vi "LaserMaster.vi"() -> ()   [LabVIEW 2014]
uses:
  Serial/Serial.lvclass
  <vilib>/Utility/file.llb/Write To Spreadsheet File (string).vi
panel:
  out "Discovery?":bool
  out "Humidity Threshold":dbl
  in  "Power (mW) 2":dbl format="%#.0f"
  out "SavePath":path
  out "Start time":timestamp
  out "Step":dbl
  out "State next step":string
  in  "stop":bool
  out "Query backup List":string[][](array[string])=[["?L", " 0\r"], ["?K", " 0\r"], ["?F", " 0\r"], ["?FH", " 2\r"], ["?SHUTTER", " 0\r"], ["?UF", " 0\r"], ["?PHLDC", " 1\r"], ["?PZTMC", " 0\r"], ["?PZTXC", " 2.24\r"], ["?PZTYC", " 2.14\r"], ["?PHLDP", " 0\r"], ["?PZTMP", " 0\r"], ["?PZTXP", " 2.58\r"], ["?PXTYP", "  Query Error:?PXTYP\r"], ["?PTRK", "  Query Error:?PTRK\r"], ["?MDLK", " 0\r"], ["?PP", " 0.80\r"], ["?TS", " 0\r"], ["?SM", " 1\r"], ["?HM", " 1\r"], ["?VW", " 850\r"], ["?STPRPOS", " 2096\r"], ["?C", " 0.00\r"], ["?D1C", " 0.08\r"], ["?D2C", " -0.43\r"], ["?BT", " 20.07\r"], ["?D1T", " 24.20\r"], ["?D2T", " 24.20\r"], ["?VT", " 20.72\r"], ["?LBOT", " 148.45\r"], ["?ET", " 39.01\r"], ["?D1ST", " 24.20\r"], ["?D2ST", " 24.20\r"], ["?VST", " 30.00\r"], ["?LBOST", " 148.41\r"], ["?EST", " 39.00\r"], ["?D1TD", " 500.12\r"], ["?D2TD", " 464.53\r"], ["?VD", " 0.00\r"], ["?LBOD", " 5358.08\r"], ["?ED", " 2152.46\r"], ["?D1HST", " 21.35\r"], ["?D2HST", " 21.48\r"], ["?LBOH", " 1\r"], ["?LRS", " 2\r"], ["?D1SS", " 1\r"], ["?D2SS", " 1\r"], ["?VSS", " 0\r"], ["?LBOSS", " 1\r"], ["?ESS", " 1\r"], ["?D1H", "  351.54\r"], ["?D2H", "  351.52\r"], ["?HH", " 37\r"], ["?D1V", " 0.19\r"], ["?D2V", " 0.18\r"], ["?SV", " 8.26,8.26,9.57\r"], ["?MB", "  Query Error:?MB\r"], ["?PI", " 2BC\r"], ["?BV", " 13.24\r"], ["?AMDLK", " 1\r"], ["?PZTS", "  Query Error:?PZTS\r"], ["?TMAX", " 1080\r"], ["?TMIN", " 680\r"], ["?ALIGN", " 0\r"], ["?ALIGNP", " 250\r"], ["?ALIGNW", " 730\r"], ["?LFP", " 0\r"], ["?PZTXCM", " 8.11\r"], ["?PZTXCP", " -10.30\r"], ["?PZTXPM", " 8.11\r"], ["?PZTXPP", " 3.06\r"], ["?PZTYCM", " 8.11\r"], ["?PZTYCP", " -14.28\r"], ["?PZTYPM", " 8.11\r"], ["?PZTYPP", " 11.74\r"], ["?RH", " 0\r"], ["?SN", " 9571\r"], ["?ST", " Standby\r"], ["?GDDCURVE", " 0\r"], ["?GDD", " 0\r"], ["?GDDCURVEN", " ZERO\r"], ["?CURVEN", " OUT OF RANGE\r"], ["?COMP", " 1\r"], ["?HMCOMP", " 1\r"], ["?GDDMAX", " 17333\r"], ["?GDDMIN", "0"]]
  out "Laser Info":i32
  out "Shutter off time":dbl
  out "Quiting":dbl
  out "Backuper state":string
  in  "Tab Control":T1(tab)
  out "Power 2":i32
  in  "Align 2":bool
  in  "Shutter 2":bool
  in  "Lock":bool
  in  "Auto":bool
  out "Baseplate Temp (C)":dbl(slide) scale=20.0..40.0
  in  "Dither hold":bool
  in  "Shutter":bool
  out "Laser Status":bool
  out "Power (mW)":dbl(knob) scale=0.0..5000.0
  out "Walking":bool
  out "Sleeping":bool
  out "ModeLocked":bool
  out "Backing up":bool
  in  "Wavelength":dbl=920.0
  in  "GDD":dbl
  in  "QUIT":bool
  out "Max":string
  in  "Align":bool
  in  "Def. Wavelength":dbl=920.0
  in  "Dither auto":dbl=120.0
  in  "Dither timer":dbl=5.0
  out "Faults":string
  in  "Home motor":bool
  in  "Optimize":bool
  in  "WV Walk":bool
  in  "Standby Time (min)":dbl=120.0
  in  "Sleep":bool
  in  "Backup":bool
  in  "Auto-Backup \nIdle Time (min)":dbl=30.0
  out "Operating Status":string
  out "Tunning Status":i32
  out "Idle Time":dbl format="%.1f"
  out "Laser On Time":dbl format="%#.1f"
  in  "Laser Control":bool
  in  "Command Line":string
  out "Laser Response":string
  in  "Refresh":bool
  out "Query List":string[][](array[string])
  out "queue #":i32
  # "LASER"
  # "LASER fine-tune"
  # "BACKUP"
  # "Timers"
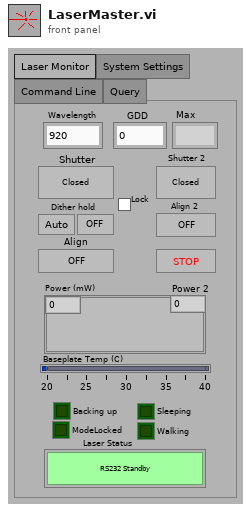
[diagram p1: front panel]
types:
  T1 = enum32{"Laser Monitor", "System Settings", "Command Line", "Query"}
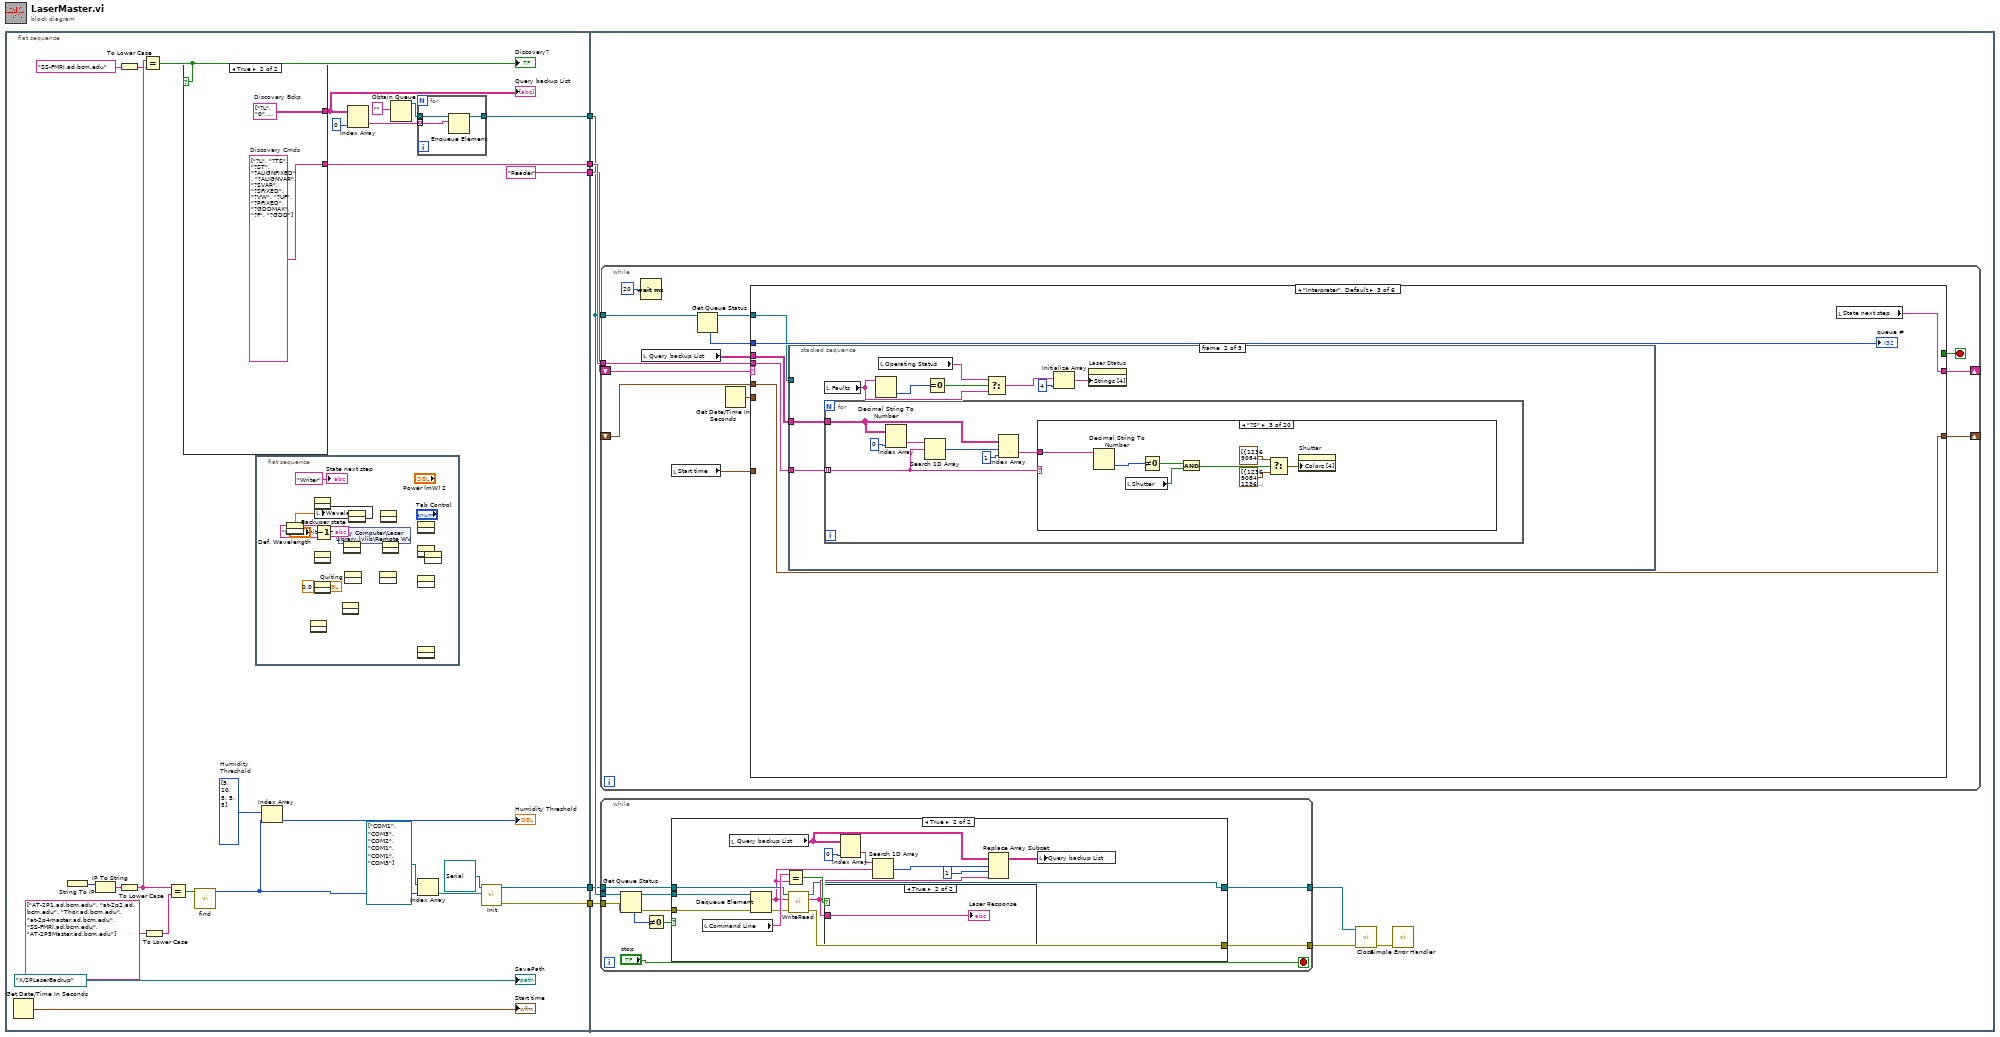
[diagram p0: block diagram]
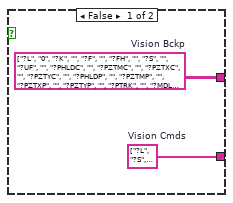
[diagram p2: hidden frame]
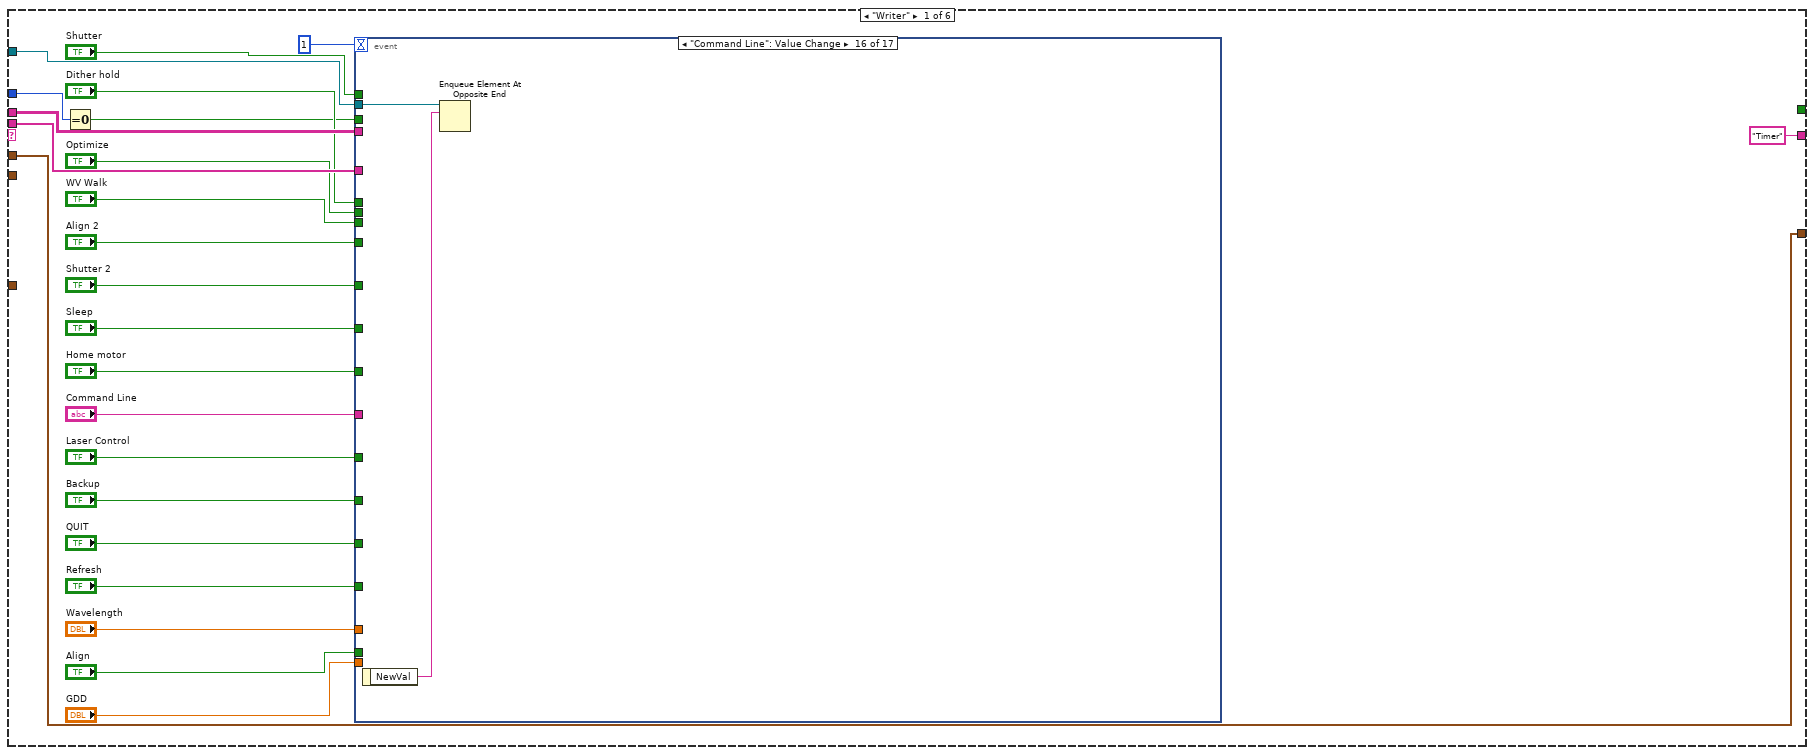
[diagram p5: hidden frame]
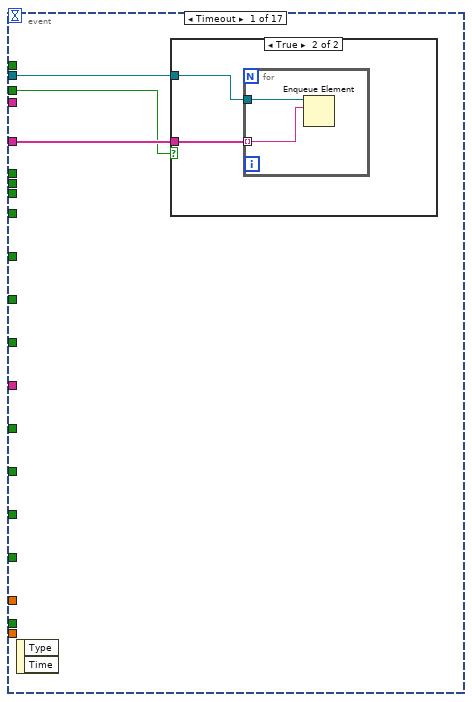
[diagram p6: hidden frame]
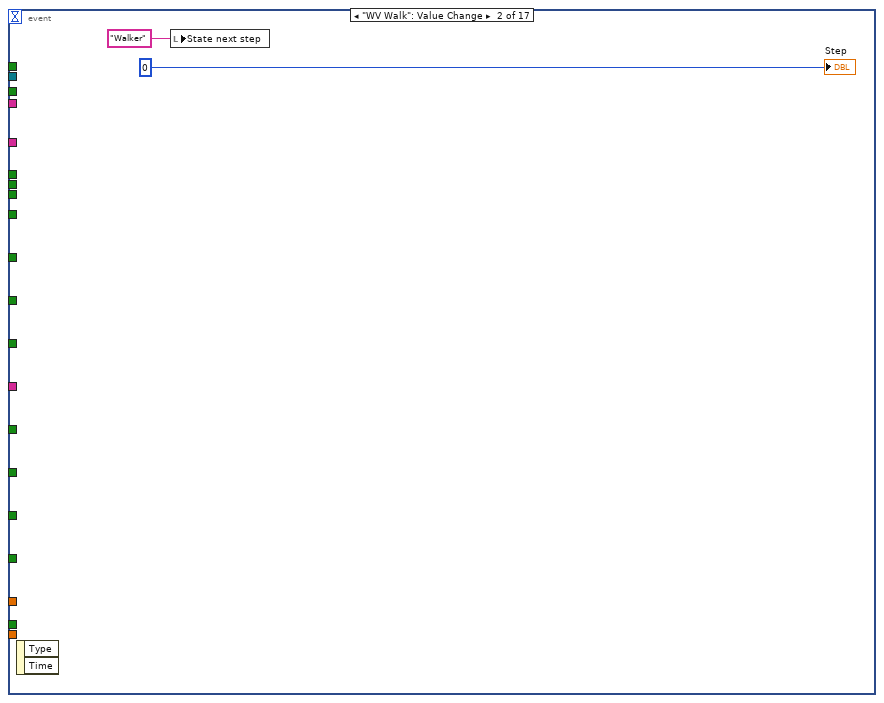
[diagram p8: hidden frame]
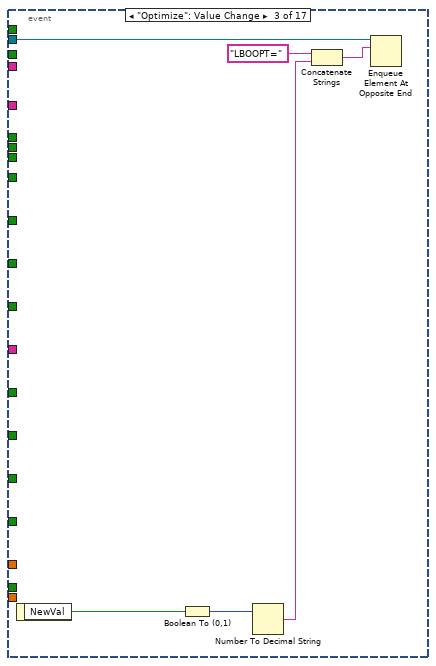
[diagram p9: hidden frame]
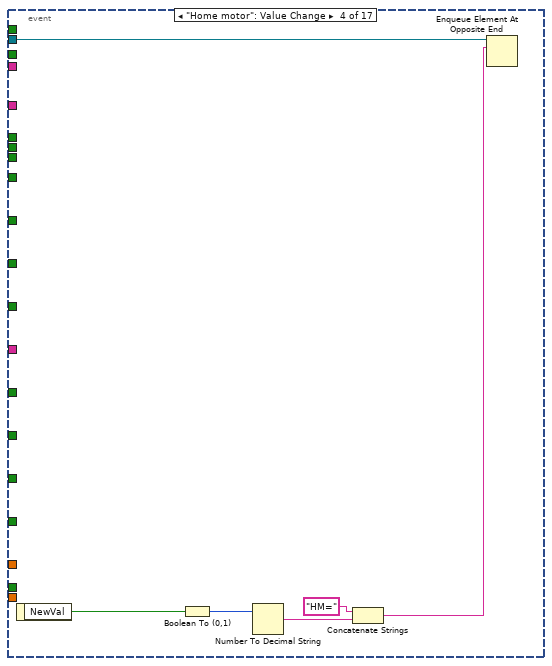
[diagram p10: hidden frame]
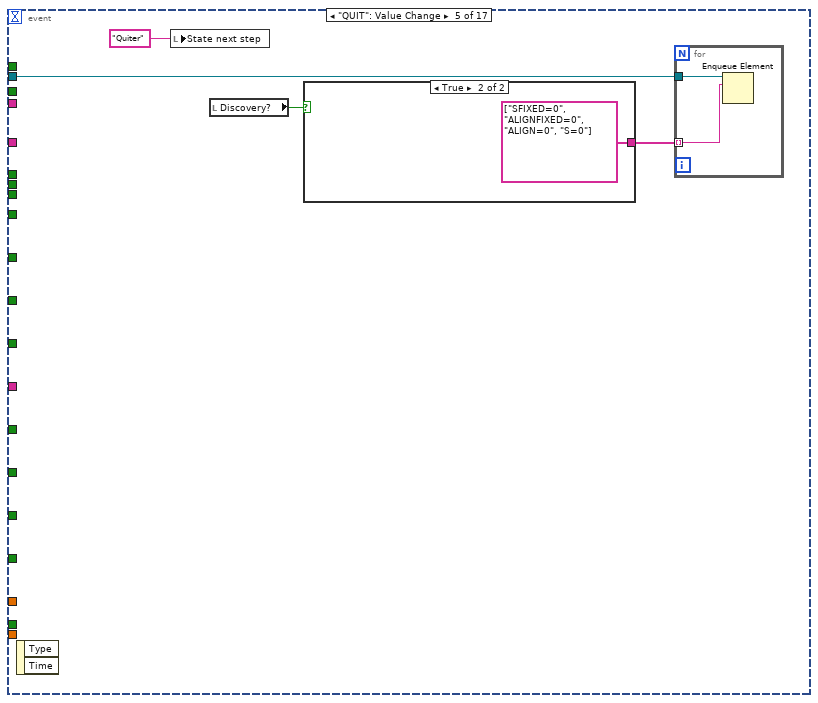
[diagram p11: hidden frame]
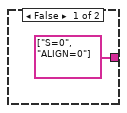
[diagram p12: hidden frame]
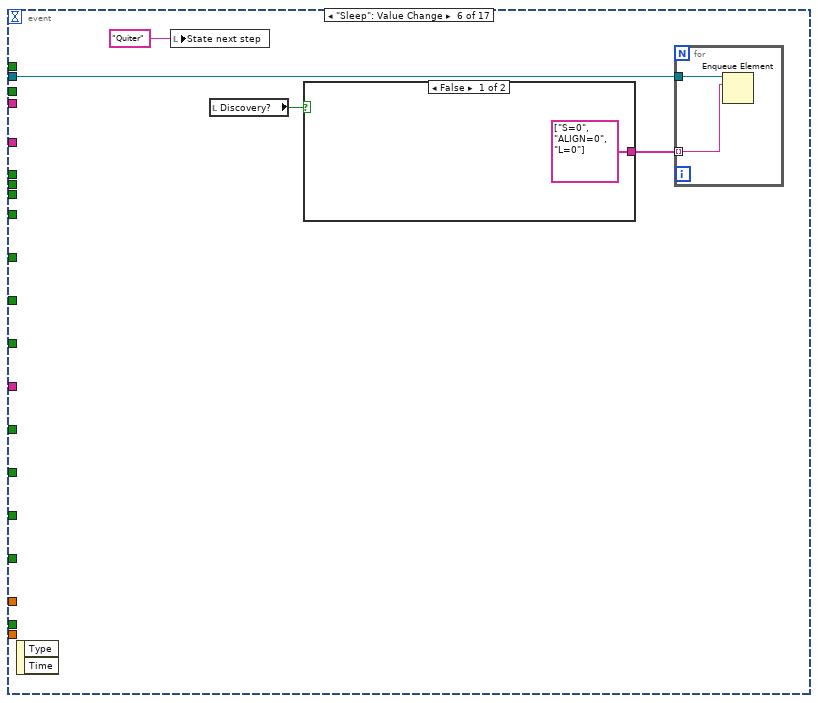
[diagram p13: hidden frame]
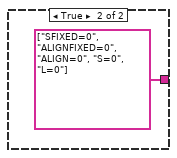
[diagram p14: hidden frame]
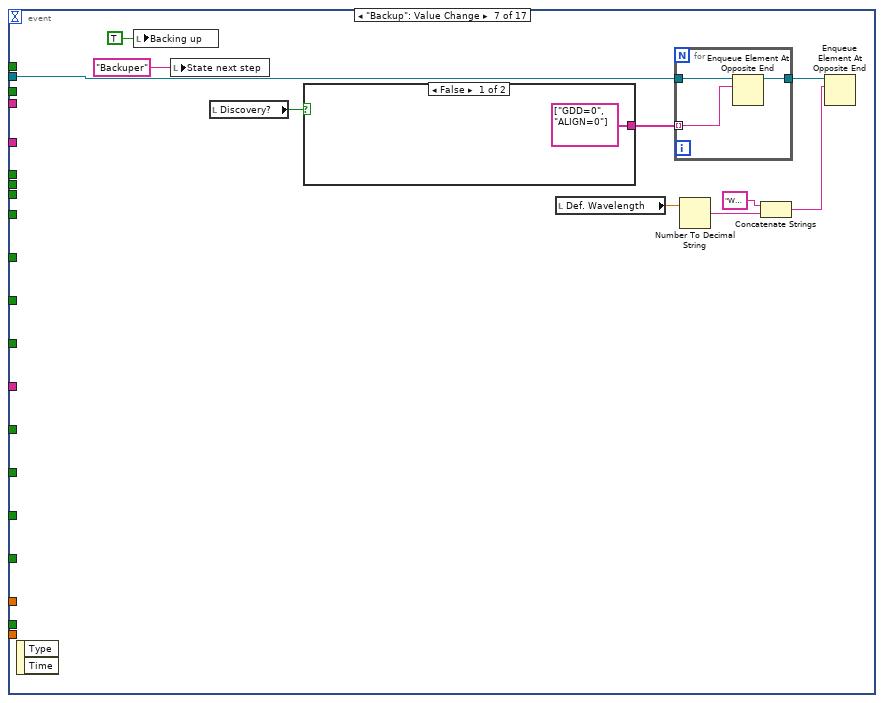
[diagram p15: hidden frame]
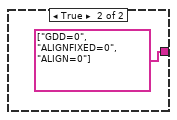
[diagram p16: hidden frame]
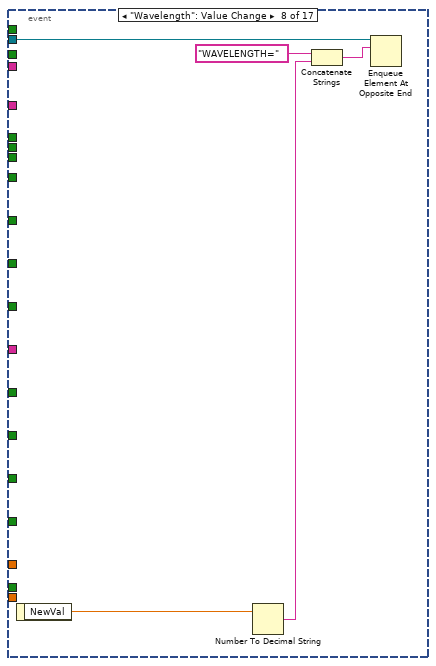
[diagram p17: hidden frame]
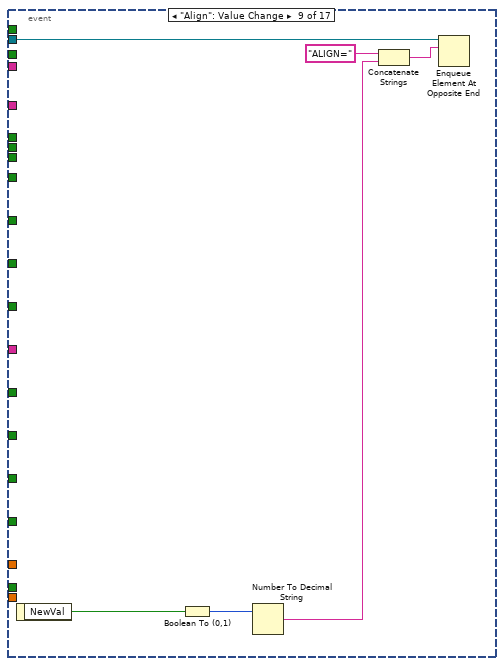
[diagram p18: hidden frame]
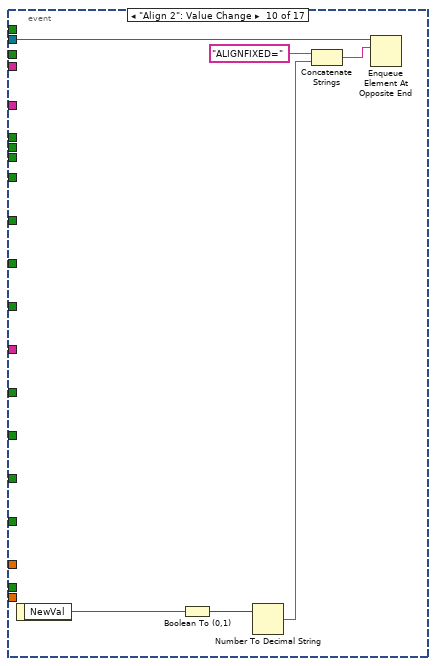
[diagram p19: hidden frame]
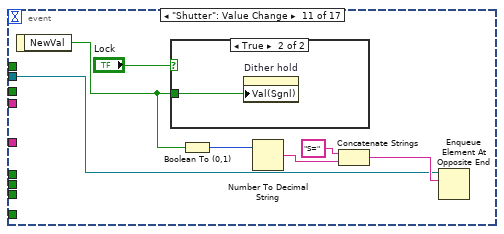
[diagram p20: hidden frame]
diagram:
  n1 = flat-sequence {
    tunnel: [w27] -> w5
    tunnel: [w10] -> w4
    tunnel: ["Reader"] -> w3
    tunnel: [w7] -> w2
    tunnel: [w6] -> w1
    tunnel: w5 -> [w50]
    tunnel: w4 -> [w52]
    tunnel: w3 -> [w51]
    tunnel: w2 -> [w49]
    tunnel: w1 -> [w48]
    frame #0 {
      w19 = i32[] [5, 10, 5, 5, 5]  # Humidity  Threshold
      n2 = Get Date/Time In Seconds() -> (seconds since 1Jan1904=→"Start time":timestamp)
      n3 = String To IP() -> (0:w24:u32)  [unwired: 1 in]
      n4 = IP To String(2:w24) -> (0:w22:string)  [unwired: 1 in]
      n5 = To Lower Case(string="SS-FMRI.ad.bcm.edu") -> (all lower case string=w13:string)
      n6 = To Lower Case(string=w22) -> (all lower case string=w15:string)
      n7 = Equal?(x=w15, y=w13) -> (x = y?=w12:bool)
      "Discovery?" <- w12
      n8 = To Lower Case(string=string[] ["AT-2P1.ad.bcm.edu", "at-2p2.ad.bcm.edu", "Thor.ad.bcm.edu", "at-2p4master.ad.bcm.edu", "SS-FMRI.ad.bcm.edu", "AT-2P5Master.ad.bcm.edu"]) -> (all lower case string=w23:string[])
      n9 = Equal?(x=w15, y=w23) -> (x = y?=w17:bool[])
      n10 = case shown="True" w12 {
        tunnel: [w34 w36] -> w11
        tunnel: [w33 w35] -> w10
        frame False {
          w33 = string[] ["?L", "?S", "?VW", "?ALIGN", "?PHLDP", "?UF", "?GDD", "?TS", "?ST", "?MDLK", "?GDDMAX", "?F", "?RH", "?BT"]  # Vision Cmds
          w34 = string[][] [["?L", "0"], ["?K", ""], ["?F", ""], ["?FH", ""], ["?S", ""], ["?UF", ""], ["?PHLDC", ""], ["?PZTMC", ""], ["?PZTXC", ""], ["?PZTYC", ""], ["?PHLDP", ""], ["?PZTMP", ""], ["?PZTXP", ""], ["?PZTYP", ""], ["?PTRK", ""], ["?MDLK", ""], ["?PP", ""], ["?TS", ""], ["?SM", ""], ["?HM", ""], ["?VW", ""], ["?STPRPOS", ""], ["?C", ""], ["?D1C", ""], ["?D2C", ""], ["?BT", ""], ["?D1T", ""], ["?D2T", ""], ["?VT", ""], ["?LBOT", ""], ["?ET", ""], ["?D1ST", ""], ["?D2ST", ""], ["?VST", ""], ["?LBOST", ""], ["?EST", ""], ["?D1TD", ""], ["?D2TD", ""], ["?VD", ""], ["?LBOD", ""], ["?ED", ""], ["?D1HST", ""], ["?D2HST", ""], ["?LBOH", ""], ["?LRS", ""], ["?D1SS", ""], ["?D2SS", ""], ["?VSS", ""], ["?LBOSS", ""], ["?ESS", ""], ["?D1H", ""], ["?D2H", ""], ["?HH", ""], ["?D1V", ""], ["?D2V", ""], ["?SV", ""], ["?PI", ""], ["?BV", ""], ["?AMDLK", ""], ["?PZTS", ""], ["?TMAX", ""], ["?TMIN", ""], ["?ALIGN", ""], ["?ALIGNP", ""], ["?ALIGNW", ""], ["?LFP", ""], ["?PZTXCM", ""], ["?PZTXCP", ""], ["?PZTXPM", ""], ["?PZTXPP", ""], ["?PZTYCM", ""], ["?PZTYCP", ""], ["?PZTYPM", ""], ["?PZTYPP", ""], ["?RH", ""], ["?SN", ""], ["?ST", ""], ["?GDDCURVE", ""], ["?GDD", ""], ["?GDDCURVEN", ""], ["?COMP", ""], ["?HMCOMP", ""], ["?GDDMAX", ""], ["?GDDMIN", ""]]  # Vision Bckp
        }
        frame True {
          w35 = string[] ["?L", "?TS", "?ST", "?ALIGNFIXED", "?ALIGNVAR", "?SVAR", "?SFIXED", "?VW", "?UF", "?PFIXED", "?GDDMAX", "?F", "?GDD"]  # Discovery Cmds
          w36 = string[][] [["?L", "0"], ["?K", ""], ["?TS", ""], ["?ST", ""], ["?ALIGNFIXED", ""], ["?ALIGNVAR", ""], ["?SVAR", ""], ["?SFIXED", ""], ["?VW", ""], ["?UF", ""], ["?PFIXED", ""], ["?HB", ""], ["?HRB", ""], ["?GDDCURVE", ""], ["?GDDCURVEN", ""], ["?GDD", ""], ["?GDDMAX", ""], ["?GDDMIN", ""], ["?SN", ""], ["?F", ""], ["?FT", ""], ["?FH", ""], ["?FHT", ""]]  # Discovery Bckp
        }
      }
      "Query backup List" <- w11
      n11 = call "find.vi"("Array"=w17) -> ("Index"=w16:i32)  [unwired: 10 in]
      n12 = flat-sequence {
        frame #0 {
          n13 = invoke on="ModeLocked" class="Bool (strict)" method="Reinit To Default"() -> ()  [unwired: 3 in, 3 out]
          n14 = invoke on="Align" class="Bool (strict)" method="Reinit To Default"() -> ()  [unwired: 3 in, 3 out]
          n15 = Decrement(x="Def. Wavelength") -> (x-1=w38:dbl)
          n16 = invoke on="Home motor" class="Bool" method="Reinit To Default"() -> ()  [unwired: 3 in, 3 out]
          n17 = invoke on="stop" class="Bool (strict)" method="Reinit To Default"() -> ()  [unwired: 3 in, 3 out]
          n18 = invoke on="Sleep" class="Bool (strict)" method="Reinit To Default"() -> ()  [unwired: 3 in, 3 out]
          n19 = local write "Wavelength"("Def. Wavelength") -> ()
          n20 = shared-variable "My Computer\\Laser Library.lvlib\\Remote WV"(w38) -> ()  [unwired: 1 in, 1 out]
          n21 = invoke on="WV Walk" class="Bool (strict)" method="Reinit To Default"() -> ()  [unwired: 3 in, 3 out]
          n22 = invoke on="Walking" class="Bool (strict)" method="Reinit To Default"() -> ()  [unwired: 3 in, 3 out]
          n23 = invoke on="Backup" class="Bool (strict)" method="Reinit To Default"() -> ()  [unwired: 3 in, 3 out]
          n24 = invoke on="Auto" class="Bool (strict)" method="Reinit To Default"() -> ()  [unwired: 3 in, 3 out]
          n25 = invoke on="Optimize" class="Bool" method="Reinit To Default"() -> ()  [unwired: 3 in, 3 out]
          n26 = invoke on="Sleeping" class="Bool (strict)" method="Reinit To Default"() -> ()  [unwired: 3 in, 3 out]
          n27 = invoke on="Refresh" class="Bool (strict)" method="Reinit To Default"() -> ()  [unwired: 3 in, 3 out]
          n28 = invoke on="Idle Time" class="DigNum (strict)" method="Reinit To Default"() -> ()  [unwired: 3 in, 3 out]
          n29 = invoke on="Laser Control" class="Bool (strict)" method="Reinit To Default"() -> ()  [unwired: 3 in, 3 out]
          n30 = invoke on="Dither hold" class="Bool (strict)" method="Reinit To Default"() -> ()  [unwired: 3 in, 3 out]
          n31 = invoke on="Backing up" class="Bool (strict)" method="Reinit To Default"() -> ()  [unwired: 3 in, 3 out]
          n32 = invoke on="QUIT" class="Bool (strict)" method="Reinit To Default"() -> ()  [unwired: 3 in, 3 out]
          "Backuper state" <- "BackupInit"
          "Quiting" <- 0.0 ("Quiting")
          "State next step" <- "Writer"
        }
      }
      n33 = Index Array(array=w19, index=w16) -> (element=→"Humidity Threshold":i32)
      n34 = Index Array(array=w11, index (col)=0 ("disabled index (col)")) -> (element=w29:string[])  [unwired: 1 in]
      n35 = Obtain Queue(element data type="") -> (queue out=w31:refnum<queue>)  [unwired: 4 in, 2 out]
      n36 = for {
        tunnel: w31 -> [w44]
        tunnel: w29 -> [w43] mode=indexing
        tunnel: [w42] -> w27
        n37 = Enqueue Element(queue=w44, element=w43) -> (queue out=w42:refnum<queue>)  [unwired: 2 in, 2 out]
      }
      n38 = Index Array(array=refnum<visa-resource-name>[] ["COM1", "COM3", "COM2", "COM1", "COM1", "COM3"], index=w16) -> (element=w9:refnum<visa-resource-name>)
      n39 = call-dynamic "Init.vi"("serial port"=w9, "Serial in"=refnum<class "Serial.lvclass"> refnum ("Serial.lvclass")) -> ("error out"=w6:errorcluster, "Serial out"=w7:refnum<class "Serial.lvclass">)  [unwired: 8 in]
      "SavePath" <- path "X:/2PLaserBackup"
    }
    frame #1 {
      n40 = while {
        tunnel: w50 -> [w91]
        tunnel: w52 -> [w92]
        shift-right: [w93] -> _
        shift-left: w51 -> [w94]
        shift-right: [w83] -> _
        shift-left: _ -> [w82]
        stop <- w88 stop-if-true
        n41 = Wait (ms)(milliseconds to wait=u32 20) -> ()  [unwired: 1 out]
        n42 = local read "Query backup List"() -> (w90:string[][])
        n43 = local read "Start time"() -> (w84:timestamp)
        n44 = Get Queue Status(queue=w91) -> (queue out=w87:refnum<queue>, # elements in queue=w86:i32)  [unwired: 2 in, 6 out]
        n45 = Get Date/Time In Seconds() -> (seconds since 1Jan1904=w85:timestamp)
        n46 = case shown="\"Interpreter\", Default" w94 {
          tunnel: w87 -> [w118 _ w298 _ _ _]
          tunnel: w90 -> [w117 _ w302 _ w495 _]
          tunnel: w92 -> [w116 _ w303 _ _ _]
          tunnel: ["Timer" "Interpreter" w301 "Writer" "Writer" w521] -> w93
          tunnel: w86 -> [w115 _ w300 _ _ w523]
          tunnel: [_ _ _ _ _ w520] -> w88
          tunnel: w85 -> [_ w232 _ _ _ _]
          tunnel: w84 -> [_ w236 _ _ _ _]
          tunnel: [w97 w233 w299 w477 w492 w519] -> w83
          tunnel: w82 -> [w97 w231 w299 w477 w492 w519]
          frame "Writer" {
            n47 = Equal To 0?(x=w115) -> (x = 0?=w103:bool)
            n48 = event shown="[15] \"Command Line\": Value Change" {
              selector: _ -> [_ _ _ _ _ _ _ _ _ _ _ _ _ _ _ _ _]
              dyn-events: _ -> [_ _ _ _ _ _ _ _ _ _ _ _ _ _ _ _ _]
              timeout: 1 -> [_ _ _ _ _ _ _ _ _ _ _ _ _ _ _ _ _]
              tunnel: w118 -> [w121 _ w128 w135 w143 w150 w165 w172 w177 w183 w190 w197 w203 w210 w215 w222 w224]
              tunnel: "Shutter" -> [_ _ _ _ _ _ _ _ _ _ _ _ _ _ _ _ _]
              tunnel: "Dither hold" -> [_ _ _ _ _ _ _ _ _ _ _ _ _ _ _ _ _]
              tunnel: "GDD" -> [_ _ _ _ _ _ _ _ _ _ _ _ _ _ _ _ _]
              tunnel: "Align" -> [_ _ _ _ _ _ _ _ _ _ _ _ _ _ _ _ _]
              tunnel: "Wavelength" -> [_ _ _ _ _ _ _ _ _ _ _ _ _ _ _ _ _]
              tunnel: "Laser Control" -> [_ _ _ _ _ _ _ _ _ _ _ _ _ _ _ _ _]
              tunnel: "Command Line" -> [_ _ _ _ _ _ _ _ _ _ _ _ _ _ _ _ _]
              tunnel: w117 -> [_ _ _ _ _ _ _ _ _ _ _ _ w202 _ _ _ _]
              tunnel: "Refresh" -> [_ _ _ _ _ _ _ _ _ _ _ _ _ _ _ _ _]
              tunnel: w116 -> [w120 _ _ _ _ _ _ _ _ _ _ _ _ _ _ _ _]
              tunnel: "QUIT" -> [_ _ _ _ _ _ _ _ _ _ _ _ _ _ _ _ _]
              tunnel: "Backup" -> [_ _ _ _ _ _ _ _ _ _ _ _ _ _ _ _ _]
              tunnel: w103 -> [w119 _ _ _ _ _ _ _ _ _ _ _ _ _ _ _ _]
              tunnel: "WV Walk" -> [_ _ _ _ _ _ _ _ _ _ _ _ _ _ _ _ _]
              tunnel: "Optimize" -> [_ _ _ _ _ _ _ _ _ _ _ _ _ _ _ _ _]
              tunnel: "Home motor" -> [_ _ _ _ _ _ _ _ _ _ _ _ _ _ _ _ _]
              tunnel: "Sleep" -> [_ _ _ _ _ _ _ _ _ _ _ _ _ _ _ _ _]
              tunnel: "Shutter 2" -> [_ _ _ _ _ _ _ _ _ _ _ _ _ _ _ _ _]
              tunnel: "Align 2" -> [_ _ _ _ _ _ _ _ _ _ _ _ _ _ _ _ _]
              event Timeout {
                n49 = event-data() -> ()  [unwired: 1 in, 2 out]
                n50 = case shown="True" w119 {
                  tunnel: w121 -> [_ w123]
                  tunnel: w120 -> [_ w122]
                  frame False {
                  }
                  frame True {
                    n51 = for {
                      tunnel: w123 -> [w125]
                      tunnel: w122 -> [w124] mode=indexing
                      n52 = Enqueue Element(queue=w125, element=w124) -> ()  [unwired: 2 in, 3 out]
                    }
                  }
                }
              }
              event "WV Walk": Value Change {
                n53 = event-data() -> ()  [unwired: 1 in, 2 out]
                n54 = local write "State next step"("Walker") -> ()
                "Step" <- 0
              }
              event "Optimize": Value Change {
                n55 = event-data() -> ("NewVal"=w129:bool)  [unwired: 1 in]
                n56 = Boolean To (0,1)(Boolean=w129) -> (0, 1=w132:i16)
                n57 = Number To Decimal String(number=w132) -> (decimal integer string=w133:string)  [unwired: 1 in]
                n58 = Concatenate Strings("LBOOPT=", w133) -> (w130:string)
                n59 = Enqueue Element At Opposite End(queue=w128, element=w130) -> ()  [unwired: 2 in, 3 out]
              }
              event "Home motor": Value Change {
                n60 = event-data() -> ("NewVal"=w134:bool)  [unwired: 1 in]
                n61 = Boolean To (0,1)(Boolean=w134) -> (0, 1=w138:i16)
                n62 = Number To Decimal String(number=w138) -> (decimal integer string=w139:string)  [unwired: 1 in]
                n63 = Concatenate Strings("HM=", w139) -> (w136:string)
                n64 = Enqueue Element At Opposite End(queue=w135, element=w136) -> ()  [unwired: 2 in, 3 out]
              }
              event "QUIT": Value Change {
                n65 = event-data() -> ()  [unwired: 1 in, 2 out]
                n66 = local write "State next step"("Quiter") -> ()
                n67 = local read "Discovery?"() -> (w140:bool)
                n68 = case shown="True" w140 {
                  tunnel: [string[] ["S=0", "ALIGN=0"] string[] ["SFIXED=0", "ALIGNFIXED=0", "ALIGN=0", "S=0"]] -> w141
                  frame False {
                  }
                  frame True {
                  }
                }
                n69 = for {
                  tunnel: w143 -> [w147]
                  tunnel: w141 -> [w146] mode=indexing
                  n70 = Enqueue Element(queue=w147, element=w146) -> ()  [unwired: 2 in, 3 out]
                }
              }
              event "Sleep": Value Change {
                n71 = event-data() -> ()  [unwired: 1 in, 2 out]
                n72 = local write "State next step"("Quiter") -> ()
                n73 = local read "Discovery?"() -> (w149:bool)
                n74 = case shown="False" w149 {
                  tunnel: [string[] ["S=0", "ALIGN=0", "L=0"] string[] ["SFIXED=0", "ALIGNFIXED=0", "ALIGN=0", "S=0", "L=0"]] -> w148
                  frame False {
                  }
                  frame True {
                  }
                }
                n75 = for {
                  tunnel: w150 -> [w155]
                  tunnel: w148 -> [w154] mode=indexing
                  n76 = Enqueue Element(queue=w155, element=w154) -> ()  [unwired: 2 in, 3 out]
                }
              }
              event "Backup": Value Change {
                n77 = event-data() -> ()  [unwired: 1 in, 2 out]
                n78 = local write "Backing up"(TRUE ("Backing up ...")) -> ()
                n79 = local write "State next step"("Backuper") -> ()
                n80 = local read "Discovery?"() -> (w157:bool)
                n81 = case shown="False" w157 {
                  tunnel: [string[] ["GDD=0", "ALIGN=0"] string[] ["GDD=0", "ALIGNFIXED=0", "ALIGN=0"]] -> w156
                  frame False {
                  }
                  frame True {
                  }
                }
                n82 = local read "Def. Wavelength"() -> (w161:dbl)
                n83 = for {
                  tunnel: w156 -> [w170] mode=indexing
                  tunnel: w165 -> [w169]
                  tunnel: [w168] -> w162
                  n84 = Enqueue Element At Opposite End(queue=w169, element=w170) -> (queue out=w168:refnum<queue>)  [unwired: 2 in, 2 out]
                }
                n85 = Number To Decimal String(number=w161) -> (decimal integer string=w159:string)  [unwired: 1 in]
                n86 = Concatenate Strings("WAVELENGTH=", w159) -> (w158:string)
                n87 = Enqueue Element At Opposite End(queue=w162, element=w158) -> ()  [unwired: 2 in, 3 out]
              }
              event "Wavelength": Value Change {
                n88 = event-data() -> ("NewVal"=w171:dbl)  [unwired: 1 in]
                n89 = Number To Decimal String(number=w171) -> (decimal integer string=w174:string)  [unwired: 1 in]
                n90 = Concatenate Strings("WAVELENGTH=", w174) -> (w175:string)
                n91 = Enqueue Element At Opposite End(queue=w172, element=w175) -> ()  [unwired: 2 in, 3 out]
              }
              event "Align": Value Change {
                n92 = event-data() -> ("NewVal"=w176:bool)  [unwired: 1 in]
                n93 = Boolean To (0,1)(Boolean=w176) -> (0, 1=w180:i16)
                n94 = Number To Decimal String(number=w180) -> (decimal integer string=w181:string)  [unwired: 1 in]
                n95 = Concatenate Strings("ALIGN=", w181) -> (w178:string)
                n96 = Enqueue Element At Opposite End(queue=w177, element=w178) -> ()  [unwired: 2 in, 3 out]
              }
              event "Align 2": Value Change {
                n97 = event-data() -> ("NewVal"=w182:bool)  [unwired: 1 in]
                n98 = Boolean To (0,1)(Boolean=w182) -> (0, 1=w186:i16)
                n99 = Number To Decimal String(number=w186) -> (decimal integer string=w187:string)  [unwired: 1 in]
                n100 = Concatenate Strings("ALIGNFIXED=", w187) -> (w184:string)
                n101 = Enqueue Element At Opposite End(queue=w183, element=w184) -> ()  [unwired: 2 in, 3 out]
              }
              event "Shutter": Value Change {
                n102 = event-data() -> ("NewVal"=w188:bool)  [unwired: 1 in]
                n103 = case shown="True" "Lock" {
                  tunnel: w188 -> [_ w195]
                  frame False {
                  }
                  frame True {
                    n104 = property on="Dither hold" class="Bool (strict)"("Val(Sgnl)"=w195) -> ()  [unwired: 2 in, 2 out]
                  }
                }
                n105 = Boolean To (0,1)(Boolean=w188) -> (0, 1=w193:i16)
                n106 = Number To Decimal String(number=w193) -> (decimal integer string=w194:string)  [unwired: 1 in]
                n107 = Concatenate Strings("S=", w194) -> (w191:string)
                n108 = Enqueue Element At Opposite End(queue=w190, element=w191) -> ()  [unwired: 2 in, 3 out]
              }
              event "Shutter 2": Value Change {
                n109 = event-data() -> ("NewVal"=w196:bool)  [unwired: 1 in]
                n110 = Boolean To (0,1)(Boolean=w196) -> (0, 1=w200:i16)
                n111 = Number To Decimal String(number=w200) -> (decimal integer string=w201:string)  [unwired: 1 in]
                n112 = Concatenate Strings("SFIXED=", w201) -> (w198:string)
                n113 = Enqueue Element At Opposite End(queue=w197, element=w198) -> ()  [unwired: 2 in, 3 out]
              }
              event "Refresh": Value Change {
                n114 = event-data() -> ()  [unwired: 1 in, 1 out]
                n115 = local write "Refresh"(FALSE ("Backup")) -> ()
                n116 = Index Array(array=w202, index (col)=0 ("disabled index (col)")) -> (element=w205:string[])  [unwired: 1 in]
                n117 = for {
                  tunnel: w203 -> [w208]
                  tunnel: w205 -> [w207] mode=indexing
                  n118 = Enqueue Element(queue=w208, element=w207) -> ()  [unwired: 2 in, 3 out]
                }
              }
              event "Dither hold": Value Change {
                n119 = event-data() -> ("NewVal"=w209:bool)  [unwired: 1 in]
                n120 = Boolean To (0,1)(Boolean=w209) -> (0, 1=w213:i16)
                n121 = Number To Decimal String(number=w213) -> (decimal integer string=w214:string)  [unwired: 1 in]
                n122 = Concatenate Strings("PHLDP=", w214) -> (w211:string)
                n123 = Enqueue Element At Opposite End(queue=w210, element=w211) -> ()  [unwired: 2 in, 3 out]
              }
              event "Laser Control": Value Change {
                n124 = event-data() -> ("NewVal"=w216:bool)  [unwired: 1 in]
                n125 = Boolean To (0,1)(Boolean=w216) -> (0, 1=w219:i16)
                n126 = Number To Decimal String(number=w219) -> (decimal integer string=w220:string)  [unwired: 1 in]
                n127 = Concatenate Strings("L=", w220) -> (w217:string)
                n128 = Enqueue Element At Opposite End(queue=w215, element=w217) -> ()  [unwired: 2 in, 3 out]
              }
              event "Command Line": Value Change {
                n129 = event-data() -> ("NewVal"=w221:string)  [unwired: 1 in]
                n130 = Enqueue Element At Opposite End(queue=w222, element=w221) -> ()  [unwired: 2 in, 3 out]
              }
              event "GDD": Value Change {
                n131 = event-data() -> ("NewVal"=w223:dbl)  [unwired: 1 in]
                n132 = Number To Decimal String(number=w223) -> (decimal integer string=w226:string)  [unwired: 1 in]
                n133 = Concatenate Strings("GDD=", w226) -> (w227:string)
                n134 = Enqueue Element At Opposite End(queue=w224, element=w227) -> ()  [unwired: 2 in, 3 out]
              }
            }
          }
          frame "Timer" {
            n135 = Subtract(x=w232, y=w236) -> (x-y=w239:dbl)
            n136 = local read "Tunning Status"() -> (w256:i32)
            n137 = local read "Laser Control"() -> (w255:bool)
            n138 = local read "Power (mW)"() -> (w229:dbl)
            n139 = case shown="True" "Auto" {
              tunnel: w232 -> [w258 w265]
              tunnel: [w258 w264] -> w233
              tunnel: w231 -> [_ w263]
              frame False {
              }
              frame True {
                n140 = Subtract(x=w265, y=w263) -> (x-y=w267:dbl)
                n141 = local read "Dither hold"() -> (w259:bool)
                n142 = Select(t="Dither auto", s=w259, f="Dither timer") -> (s? t:f=w260:dbl)
                n143 = Greater?(x=w267, y=w260) -> (0:w266:bool)
                n144 = case shown="True" w266 {
                  tunnel: w265 -> [_ w271]
                  tunnel: [w268 w271] -> w264
                  tunnel: w263 -> [w268 _]
                  tunnel: w259 -> [_ w270]
                  frame False {
                  }
                  frame True {
                    n145 = Not(x=w270) -> (.not. x?=w269:bool)
                    n146 = property on="Dither hold" class="Bool (strict)"("Val(Sgnl)"=w269) -> ()  [unwired: 2 in, 2 out]
                  }
                }
              }
            }
            n147 = Not(x=w255) -> (.not. x?=w251:bool)
            n148 = Equal To 0?(x=w256) -> (x = 0?=w250:bool)
            n149 = Less?(x=w229, y=1.0) -> (x < y?=w228:bool)
            n150 = local read "Shutter off time"() -> (w246:dbl)
            n151 = local read "Shutter"() -> (w247:bool)
            n152 = Compound Arithmetic op=AND(w228, w251, w250) -> (w252:bool)
            n153 = Divide(x=w239, y=60.0 ("x")) -> (x/y=w237:dbl)
            n154 = case shown="False" w252 {
              tunnel: [w272 w283] -> w249
              tunnel: [w276 w283] -> w248
              tunnel: w247 -> [w275 _]
              tunnel: w246 -> [w274 _]
              tunnel: [w273 w283] -> w245
              tunnel: w237 -> [w272 _]
              frame False {
                n155 = case shown="False" w275 {
                  tunnel: [w279 0] -> w276
                  tunnel: w272 -> [w278 w280]
                  tunnel: w274 -> [w277 _]
                  tunnel: [w277 w280] -> w273
                  frame False {
                    n156 = Subtract(x=w278, y=w277) -> (x-y=w279:dbl)
                  }
                  frame True {
                  }
                }
              }
              frame True {
                w283 = 0
                n157 = Get Date/Time In Seconds() -> (seconds since 1Jan1904=w282:timestamp)
                n158 = local write "Start time"(w282) -> ()
              }
            }
            "Laser On Time" <- w249
            "Idle Time" <- w248
            "Shutter off time" <- w245
            n159 = local read "Backing up"() -> (w240:bool)
            n160 = Greater?(x=w248, y="Auto-Backup \nIdle Time (min)") -> (0:w243:bool)
            n161 = Greater?(x=w248, y="Standby Time (min)") -> (0:w235:bool)
            n162 = Not(x=w240) -> (.not. x?=w242:bool)
            n163 = case shown="True" w235 {
              tunnel: [FALSE ("Sleeping") w285] -> w244
              frame False {
              }
              frame True {
                w285 = TRUE
                n164 = property on="Sleep" class="Bool (strict)"("Val(Sgnl)"=w285) -> ()  [unwired: 2 in, 2 out]
              }
            }
            "Sleeping" <- w244
            n165 = And(x=w243, y=w242) -> (x .and. y?=w241:bool)
            n166 = case shown="True" w241 {
              frame False {
              }
              frame True {
                n167 = Get Date/Time In Seconds() -> (seconds since 1Jan1904=w292:timestamp)
                n168 = Format Date/Time String(time format string (%c)="%Y-%m-%d-*", seconds (now)=w292) -> (date/time string=w289:string)  [unwired: 1 in]
                n169 = String To IP() -> (0:w290:u32)  [unwired: 1 in]
                n170 = local read "SavePath"() -> (w286:path)
                n171 = IP To String(2:w290) -> (0:w287:string)  [unwired: 1 in]
                n172 = Concatenate Strings(w289, ".csv" ("string")) -> (w294:string)
                n173 = call "create unique folder.vi"("string"=w287, "path 2"=w286) -> ("path"=w295:path)  [unwired: 9 in]
                n174 = call <vilib>:"Recursive File List.vi"("pattern"=w294, "Folder Path"=w295) -> ("Number of Files"=w296:i32)  [unwired: 5 in, 4 out]
                n175 = Equal To 0?(x=w296) -> (x = 0?=w288:bool)
                n176 = case shown="True" w288 {
                  frame False {
                  }
                  frame True {
                    n177 = property on="Backup" class="Bool (strict)"("Val(Sgnl)"=TRUE) -> ()  [unwired: 2 in, 2 out]
                  }
                }
              }
            }
          }
          frame "Interpreter", Default {
            n178 = stacked-sequence {
              tunnel: w303 -> [_ w318 _ _ _]
              tunnel: w302 -> [_ w317 _ w442 _]
              tunnel: w298 -> [w304 _ _ _ _]
              frame #0 {
                n179 = local read "Command Line"() -> (w306:string)
                n180 = feedback-in #1(w306) -> ()
                n181 = feedback #1() -> (w307:string)  [unwired: 1 in]
                n182 = Not Equal?(x=w307, y=w306) -> (x != y?=w305:bool)
                n183 = case shown="True" w305 {
                  tunnel: w304 -> [_ w309]
                  tunnel: w306 -> [_ w308]
                  frame False {
                  }
                  frame True {
                    n184 = Enqueue Element At Opposite End(queue=w309, element=w308) -> ()  [unwired: 2 in, 3 out]
                  }
                }
              }
              frame #1 {
                n185 = local read "Faults"() -> (w311:string)
                n186 = for {
                  tunnel: w318 -> [w320] mode=indexing
                  tunnel: w317 -> [w321]
                  n187 = Index Array(array=w321, index (col)=0 ("disabled index (col)")) -> (element=w324:string[])  [unwired: 1 in]
                  n188 = Search 1D Array(1D array=w324, element=w320) -> (index of element=w322:i32)  [unwired: 1 in]
                  n189 = Index Array(array=w321, index (row)=w322, index (col)=1 ("disabled index (col)")) -> (element=w319:string)
                  n190 = case shown="\"?S\"" w320 {
                    tunnel: w319 -> [_ w326 w332 w337 w342 w350 w358 w366 w374 w378 w387 w390 w392 w400 w402 w404 w406 w407 w418 w420]
                    frame "False", Default {
                    }
                    frame "?L" {
                      n191 = Decimal String To Number(string=w326) -> (number=→"Laser Info":i32)  [unwired: 2 in, 1 out]
                    }
                    frame "?S" {
                      n192 = Decimal String To Number(string=w332) -> (number=w333:i32)  [unwired: 2 in, 1 out]
                      n193 = local read "Shutter"() -> (w335:bool)
                      n194 = Not Equal To 0?(x=w333) -> (x != 0?=w334:bool)
                      n195 = And(x=w334, y=w335) -> (x .and. y?=w328:bool)
                      n196 = Select(t=cluster{u32, u32}[] [{12369084, 12369084}, {6618880, 6618880}] ("Colors [4]"), s=w328, f=cluster{u32, u32}[] [{12369084, 12369084}, {12369084, 12369084}] ("Colors [4]")) -> (s? t:f=w329:cluster{u32, u32}[])
                      n197 = property on="Shutter" class="Bool (strict)"("Colors [4]"=w329) -> ()  [unwired: 2 in, 2 out]
                    }
                    frame "?VW" {
                      n198 = Decimal String To Number(string=w337) -> (number=w336:i32)  [unwired: 2 in, 1 out]
                      n199 = property on="Wavelength" class="DigNum (strict)"("Value"=w336) -> ()  [unwired: 2 in, 2 out]
                      n200 = shared-variable ".\\Laser Library.lvlib\\WV"(w336) -> ()  [unwired: 1 in, 1 out]
                    }
                    frame "?SVAR" {
                      n201 = Decimal String To Number(string=w342) -> (number=w343:i32)  [unwired: 2 in, 1 out]
                      n202 = local read "Shutter"() -> (w345:bool)
                      n203 = Not Equal To 0?(x=w343) -> (x != 0?=w344:bool)
                      n204 = And(x=w344, y=w345) -> (x .and. y?=w338:bool)
                      n205 = Select(t=cluster{u32, u32}[] [{12369084, 12369084}, {6618880, 6618880}] ("Colors [4]"), s=w338, f=cluster{u32, u32}[] [{12369084, 12369084}, {12369084, 12369084}] ("Colors [4]")) -> (s? t:f=w339:cluster{u32, u32}[])
                      n206 = property on="Shutter" class="Bool (strict)"("Colors [4]"=w339) -> ()  [unwired: 2 in, 2 out]
                    }
                    frame "?SFIXED" {
                      n207 = Decimal String To Number(string=w350) -> (number=w351:i32)  [unwired: 2 in, 1 out]
                      n208 = local read "Shutter 2"() -> (w353:bool)
                      n209 = Not Equal To 0?(x=w351) -> (x != 0?=w352:bool)
                      n210 = And(x=w352, y=w353) -> (x .and. y?=w346:bool)
                      n211 = Select(t=cluster{u32, u32}[] [{12369084, 12369084}, {6618880, 6618880}] ("Colors [4]"), s=w346, f=cluster{u32, u32}[] [{12369084, 12369084}, {12369084, 12369084}] ("Colors [4]")) -> (s? t:f=w349:cluster{u32, u32}[])
                      n212 = property on="Shutter 2" class="Bool (strict)"("Colors [4]"=w349) -> ()  [unwired: 2 in, 2 out]
                    }
                    frame "?ALIGN" {
                      n213 = Decimal String To Number(string=w358) -> (number=w359:i32)  [unwired: 2 in, 1 out]
                      n214 = Not Equal To 0?(x=w359) -> (x != 0?=w361:bool)
                      n215 = local read "Align"() -> (w360:bool)
                      n216 = And(x=w361, y=w360) -> (x .and. y?=w355:bool)
                      n217 = Select(t=cluster{u32, u32}[] [{12369084, 12369084}, {6618880, 6618880}] ("Colors [4]"), s=w355, f=cluster{u32, u32}[] [{12369084, 12369084}, {12369084, 12369084}] ("Colors [4]")) -> (s? t:f=w354:cluster{u32, u32}[])
                      n218 = property on="Align" class="Bool (strict)"("Colors [4]"=w354) -> ()  [unwired: 2 in, 2 out]
                    }
                    frame "?ALIGNVAR" {
                      n219 = Decimal String To Number(string=w366) -> (number=w367:i32)  [unwired: 2 in, 1 out]
                      n220 = Not Equal To 0?(x=w367) -> (x != 0?=w369:bool)
                      n221 = local read "Align"() -> (w368:bool)
                      n222 = And(x=w369, y=w368) -> (x .and. y?=w362:bool)
                      n223 = Select(t=cluster{u32, u32}[] [{12369084, 12369084}, {6618880, 6618880}] ("Colors [4]"), s=w362, f=cluster{u32, u32}[] [{12369084, 12369084}, {12369084, 12369084}] ("Colors [4]")) -> (s? t:f=w363:cluster{u32, u32}[])
                      n224 = property on="Align" class="Bool (strict)"("Colors [4]"=w363) -> ()  [unwired: 2 in, 2 out]
                    }
                    frame "?ALIGNFIXED" {
                      n225 = Decimal String To Number(string=w374) -> (number=w375:i32)  [unwired: 2 in, 1 out]
                      n226 = local read "Align 2"() -> (w376:bool)
                      n227 = Not Equal To 0?(x=w375) -> (x != 0?=w377:bool)
                      n228 = And(x=w377, y=w376) -> (x .and. y?=w371:bool)
                      n229 = Select(t=cluster{u32, u32}[] [{12369084, 12369084}, {6618880, 6618880}] ("Colors [4]"), s=w371, f=cluster{u32, u32}[] [{12369084, 12369084}, {12369084, 12369084}] ("Colors [4]")) -> (s? t:f=w372:cluster{u32, u32}[])
                      n230 = property on="Align 2" class="Bool (strict)"("Colors [4]"=w372) -> ()  [unwired: 2 in, 2 out]
                    }
                    frame "?PHLDP" {
                      n231 = Decimal String To Number(string=w378) -> (number=w379:i32)  [unwired: 2 in, 1 out]
                      n232 = Not Equal To 0?(x=w379) -> (x != 0?=w382:bool)
                      n233 = local read "Dither hold"() -> (w380:bool)
                      n234 = And(x=w382, y=w380) -> (x .and. y?=w381:bool)
                      n235 = case shown="False" w381 {
                        frame False {
                          n236 = property on="Dither hold" class="Bool (strict)"("Colors [4]"=cluster{u32, u32}[] [{12369084, 12369084}, {12369084, 12369084}]) -> ()  [unwired: 2 in, 2 out]
                        }
                        frame True {
                          n237 = property on="Dither hold" class="Bool (strict)"("Colors [4]"=cluster{u32, u32}[] [{12369084, 12369084}, {6618880, 6618880}]) -> ()  [unwired: 2 in, 2 out]
                        }
                      }
                    }
                    frame "?UF" {
                      n238 = Decimal String To Number(string=w387) -> (number=w386:i32)  [unwired: 2 in, 1 out]
                      n239 = Round To Nearest(number=w386) -> (nearest integer value=→"Power (mW)":i32)
                    }
                    frame "?PFIXED" {
                      n240 = Decimal String To Number(string=w390) -> (number=w389:i32)  [unwired: 2 in, 1 out]
                      n241 = Round To Nearest(number=w389) -> (nearest integer value=→"Power 2":i32)
                    }
                    frame "?GDD" {
                      n242 = Decimal String To Number(string=w392) -> (number=w391:i32)  [unwired: 2 in, 1 out]
                      n243 = property on="GDD" class="DigNum (strict)"("Value"=w391) -> ()  [unwired: 2 in, 2 out]
                      n244 = shared-variable "My Computer\\Laser Library.lvlib\\GDD"(w391) -> ()  [unwired: 1 in, 1 out]
                    }
                    frame "?GDDMAX" {
                      n245 = Decimal String To Number(string=w400) -> (number=w398:i32)  [unwired: 2 in, 1 out]
                      n246 = Divide(x=w398, y=1000.0) -> (x/y=w394:dbl)
                      n247 = Round To Nearest(number=w394) -> (nearest integer value=w393:dbl)
                      n248 = Number To Decimal String(number=w393) -> (decimal integer string=w397:string)  [unwired: 1 in]
                      n249 = Concatenate Strings(w397, "k" ("string")) -> (→"Max":string)
                    }
                    frame "?TS" {
                      n250 = Decimal String To Number(string=w402) -> (number=→"Tunning Status":i32)  [unwired: 2 in, 1 out]
                    }
                    frame "?MDLK" {
                      n251 = Decimal String To Number(string=w404) -> (number=w405:i32)  [unwired: 2 in, 1 out]
                      n252 = Not Equal To 0?(x=w405) -> (x != 0?=→"ModeLocked":bool)
                    }
                    frame "?ST" {
                      "Operating Status" <- w406
                    }
                    frame "?F" {
                      "Faults" <- w407
                    }
                    frame "?RH" {
                      n253 = Decimal String To Number(string=w418) -> (number=w417:i32)  [unwired: 2 in, 1 out]
                      n254 = local read "Humidity Threshold"() -> (w408:dbl)
                      n255 = local read "Operating Status"() -> (w411:string)
                      n256 = local read "Laser Info"() -> (w414:i32)
                      n257 = Concatenate Strings(w411, "\nHigh Humidity") -> (w409:string)
                      n258 = Greater?(x=w417, y=w408) -> (0:w416:bool)
                      n259 = Select(t=w409, s=w416, f=w411) -> (s? t:f=w412:string)
                      n260 = Select(t=2, s=w416, f=w414) -> (s? t:f=w415:i32)
                      n261 = local write "Operating Status"(w412) -> ()
                      n262 = local write "Laser Info"(w415) -> ()
                    }
                    frame "?BT" {
                      n263 = Decimal String To Number(string=w420) -> (number=→"Baseplate Temp (C)":i32)  [unwired: 2 in, 1 out]
                    }
                  }
                }
                n264 = Decimal String To Number(string=w311) -> (number=w312:i32)  [unwired: 2 in, 1 out]
                n265 = local read "Operating Status"() -> (w313:string)
                n266 = Equal To 0?(x=w312) -> (x = 0?=w310:bool)
                n267 = Select(t=w313, s=w310, f=w311) -> (s? t:f=w314:string)
                n268 = Initialize Array(w314, 4 ("dimension size")) -> (w315:string[])
                n269 = property on="Laser Status" class="Bool (strict)"("Strings [4]"=w315) -> ()  [unwired: 2 in, 2 out]
              }
              frame #2 {
                n270 = local read "Tunning Status"() -> (w425:i32)
                n271 = local read "Laser Info"() -> (w423:i32)
                n272 = Equal To 0?(x=w425) -> (x = 0?=w426:bool)
                n273 = Equal To 0?(x=w423) -> (x = 0?=w422:bool)
                n274 = And(x=w426, y=w422) -> (x .and. y?=w424:bool)
                n275 = Equal?(x=w423, y=2.0) -> (x = y?=w428:bool)
                n276 = case shown="False" w428 {
                  tunnel: w424 -> [w430 _]
                  tunnel: [w429 cluster{u32, u32}[] [{16723218, 15670016}, {16721170, 16725034}] ("Colors [4]")] -> w421
                  frame False {
                    n277 = case shown="False" w430 {
                      tunnel: [w431 cluster{u32, u32}[] [{10682272, 10682272}, {12451729, 12451729}] ("Colors [4]")] -> w429
                      frame False {
                        w436 = TRUE ("Laser Status")
                        n278 = local read "Operating Status"() -> (w435:string)
                        n279 = local write "Laser Control"(w436) -> ()
                        n280 = local write "Laser Status"(w436) -> ()
                        n281 = Equal?(x=w435, y="OK") -> (x = y?=w432:bool)
                        n282 = Select(t=cluster{u32, u32}[] [{6618880, 6618880}] ("Colors [4]"), s=w432, f=cluster{u32, u32}[] [{16762130, 16762130}, {10441728, 10441728}, {10441728, 10441728}] ("Colors [4]")) -> (s? t:f=w431:cluster{u32, u32}[])
                      }
                      frame True {
                        w439 = FALSE
                        n283 = local write "Laser Control"(w439) -> ()
                        "Laser Status" <- w439
                      }
                    }
                  }
                  frame True {
                  }
                }
                n284 = property on="Laser Status" class="Bool (strict)"("Colors [4]"=w421) -> ()  [unwired: 2 in, 2 out]
              }
              frame #3 {
                w444 = 2.0 ("y")
                w447 = 30
                n285 = Array Size(array=w442) -> (size(s)=w458:i32[])
                n286 = Index Array(array=w458, index=0) -> (element=w455:i32)
                n287 = Index Array(array=w458, index=1) -> (element=w454:i32)
                n288 = Multiply(x=w455, y=w454) -> (x*y=w452:i32)
                n289 = Divide(x=w452, y=w447) -> (x/y=w453:dbl)
                n290 = Divide(x=w447, y=w444) -> (x/y=w448:dbl)
                n291 = Reshape Array(w442, w452) -> (w451:string[])
                n292 = Subtract(x=w444, y=2.0) -> (x-y=w445:dbl)
                n293 = Round Toward +Infinity(x=w453) -> (ceil(x): smallest int >= x=w446:dbl)
                n294 = Initialize Array("", w448, w445) -> (w449:string[][])
                n295 = for {
                  N: w446 -> [_]
                  tunnel: w447 -> [w472]
                  shift-right: [w470] -> _
                  shift-left: w451 -> [w471]
                  tunnel: w447 -> [w466]
                  tunnel: w444 -> [w459]
                  shift-right: [w460] -> w441
                  shift-left: w449 -> [w462]
                  i -> [w469]
                  n296 = Divide(x=w466, y=w459) -> (x/y=w465:dbl)
                  n297 = Multiply(x=w469, y=w459) -> (x*y=w461:dbl)
                  n298 = Round Toward -Infinity(1:w465) -> (0:w464:dbl)
                  n299 = Split 1D Array(array=w471, index=w472) -> (first subarray=w468:string[], second subarray=w470:string[])
                  n300 = Reshape Array(w468, w464, 2 ("dimension size")) -> (w463:string[][])
                  n301 = Insert Into Array(array=w462, index (col)=w461, new element=w463) -> (w460:string[][])  [unwired: 1 in]
                }
                "Query List" <- w441
              }
              frame #4 {
                n302 = shared-variable ".\\Laser Library.lvlib\\Remote WV"() -> (w473:dbl)  [unwired: 1 in, 1 out]
                n303 = feedback-in #2(w473) -> ()
                n304 = feedback #2(w473) -> (w475:dbl)
                n305 = Not Equal?(x=w473, y=w475) -> (x != y?=w474:bool)
                n306 = case shown="True" w474 {
                  tunnel: w473 -> [_ w476]
                  frame False {
                  }
                  frame True {
                    n307 = property on="Wavelength" class="DigNum (strict)"("Val(Sgnl)"=w476) -> ()  [unwired: 2 in, 2 out]
                  }
                }
              }
            }
            n308 = local read "State next step"() -> (w301:string)
            "queue #" <- w300
          }
          frame "Walker" {
            w483 = dbl[] [680.0, 730.0, 780.0, 830.0, 880.0, 930.0, 980.0, 1030.0, 980.0, 930.0, 880.0, 830.0, 780.0, 730.0, 680.0, 800.0] ("Array")
            n309 = Wait (ms)(milliseconds to wait=2000) -> ()  [unwired: 1 out]
            n310 = local read "Step"() -> (w485:dbl)
            n311 = Index Array(array=w483, index=w485) -> (element=w479:dbl)
            n312 = Array Size(array=w483) -> (size(s)=w482:i32)
            n313 = Increment(x=w485) -> (x+1=w481:dbl)
            n314 = property on="Wavelength" class="DigNum (strict)"("Val(Sgnl)"=w479) -> ()  [unwired: 2 in, 2 out]
            n315 = Equal?(x=w481, y=w482) -> (x = y?=w480:bool)
            n316 = case shown="True" w480 {
              tunnel: w481 -> [w488 _]
              tunnel: [TRUE FALSE ("Walking")] -> w478
              frame False {
                n317 = local write "Step"(w488) -> ()
              }
              frame True {
                n318 = local write "WV Walk"(FALSE) -> ()
                n319 = local write "State next step"("Writer") -> ()
              }
            }
            "Walking" <- w478
          }
          frame "Backuper" {
            n320 = local read "Backuper state"() -> (w493:string)
            n321 = case shown="\"BackupFinal\"" w493 {
              tunnel: w495 -> [_ w518]
              frame "BackupInit", Default {
                n322 = flat-sequence {
                  frame #0 {
                    n323 = Wait (ms)(milliseconds to wait=u32 30000) -> ()  [unwired: 1 out]
                    n324 = local write "Backuper state"("BackupFinal") -> ()
                  }
                  frame #1 {
                    n325 = local write "Refresh"(TRUE ("Refresh")) -> ()
                  }
                }
              }
              frame "BackupFinal" {
                n326 = local write "Backup"(FALSE ("Backup")) -> ()
                n327 = local write "State next step"("Writer") -> ()
                n328 = local write "Backuper state"("BackupInit") -> ()
                n329 = String To IP() -> (0:w512:u32)  [unwired: 1 in]
                n330 = local read "SavePath"() -> (w499:path)
                n331 = IP To String(2:w512) -> (0:w500:string)  [unwired: 1 in]
                n332 = call "create unique folder.vi"("string"=w500, "path 2"=w499) -> ("path"=w505:path)  [unwired: 9 in]
                n333 = Get Date/Time In Seconds() -> (seconds since 1Jan1904=w514:timestamp)
                n334 = Format Date/Time String(time format string (%c)="%Y-%m-%d-%H-%M-%S", seconds (now)=w514) -> (date/time string=w509:string)  [unwired: 1 in]
                n335 = Path To String(path=w505) -> (string=w511:string)
                n336 = Concatenate Strings(w511, "\\" ("string"), w509, ".csv" ("string")) -> (w508:string)
                n337 = String To Path(string=w508) -> (path=w507:path)
                n338 = call-poly <vilib>:"Write To Spreadsheet File.vi"("delimiter (\\t)"="," ("delimiter (\\t)"), "format (%s)"="%.6f" ("format (%.3f)"), "append to file? (new file:F)"=FALSE, "2D data"=w518, "file path (dialog if empty)"=w507) -> ()  [unwired: 2 in, 2 out]
                "Backing up" <- FALSE ("Backing up ...")
              }
            }
          }
          frame "Quiter" {
            n339 = Equal To 0?(x=w523) -> (x = 0?=w522:bool)
            n340 = case shown="True" w522 {
              tunnel: ["Quiter" "Writer"] -> w521
              tunnel: [FALSE w527] -> w520
              frame False {
              }
              frame True {
                n341 = local read "Sleep"() -> (w526:bool)
                n342 = case shown="True" w526 {
                  tunnel: [w530 _] -> w527
                  frame False {
                    n343 = local read "QUIT"() -> (w529:bool)
                    n344 = case shown="True" w529 {
                      tunnel: [_ w531] -> w530
                      frame False {
                      }
                      frame True {
                        w531 = TRUE
                        n345 = local write "QUIT"(FALSE) -> ()
                        n346 = local write "stop"(w531) -> ()
                      }
                    }
                  }
                  frame True {
                    w533 = FALSE ("Sleep")
                    n347 = local write "State next step"("Writer" ("State next step")) -> ()
                    n348 = local write "Sleep"(w533) -> ()
                    n349 = local write "Sleeping"(w533) -> ()
                    n350 = property on="Laser Control" class="Bool (strict)"("Val(Sgnl)"=w533) -> ()  [unwired: 2 in, 2 out]
                  }
                }
              }
            }
          }
        }
      }
      n351 = while {
        tunnel: w50 -> [w61]
        tunnel: w49 -> [w57]
        tunnel: w48 -> [w53]
        tunnel: [w56] -> w47
        tunnel: [w55] -> w46
        stop <- "stop" stop-if-true
        n352 = Get Queue Status(queue=w61, error in (no error)=w53) -> (queue out=w58:refnum<queue>, error out=w54:errorcluster, # elements in queue=w60:i32)  [unwired: 1 in, 5 out]
        n353 = Not Equal To 0?(x=w60) -> (x != 0?=w59:bool)
        n354 = case shown="True" w59 {
          tunnel: w58 -> [_ w76]
          tunnel: w57 -> [w63 w71]
          tunnel: [w63 w68] -> w56
          tunnel: [w64 w67] -> w55
          tunnel: w54 -> [w64 w66]
          frame False {
          }
          frame True {
            n355 = local read "Command Line"() -> (w73:string)
            n356 = local read "Query backup List"() -> (w75:string[][])
            n357 = Dequeue Element(queue=w76, error in (no error)=w66) -> (element=w70:string, error out=w65:errorcluster)  [unwired: 1 in, 2 out]
            n358 = Equal?(x=w73, y=w70) -> (x = y?=w72:bool)
            n359 = call-dynamic "WriteRead.vi"("error in (no error)"=w65, "Command"=w70, "Serial in"=w71) -> ("error out"=w67:errorcluster, "Response"=w69:string, "Serial out"=w68:refnum<class "Serial.lvclass">)  [unwired: 6 in]
            n360 = case shown="True" w72 {
              tunnel: w69 -> [_ w81]
              frame False {
              }
              frame True {
                "Laser Response" <- w81
              }
            }
            n361 = Index Array(array=w75, index (col)=0 ("index (row)")) -> (element=w79:string[])  [unwired: 1 in]
            n362 = Search 1D Array(1D array=w79, element=w70) -> (index of element=w77:i32)  [unwired: 1 in]
            n363 = Replace Array Subset(array=w75, new element=w69, index (row)=w77, index (col)=1 ("disabled index (col)")) -> (w74:string[][])
            n364 = local write "Query backup List"(w74) -> ()
          }
        }
      }
      n365 = call-dynamic "Close.vi"("error in (no error)"=w46, "Serial in"=w47) -> ("error out"=w45:errorcluster)  [unwired: 8 in, 1 out]
      n366 = call <vilib>:"Simple Error Handler.vi"("error in (no error)"=w45) -> ()  [unwired: 1 in, 8 out]
    }
  }
